vi "Thermo Analyzers Example 1.vi"() -> ()   [LabVIEW 2012]
uses:
  <vilib>/Analysis/Matrix/Datatypes/RealMatrix.ctl
  <vilib>/Analysis/Matrix/NI_Matrix.lvlib
panel:
  in  "Frequency (Hz)":dbl=0.1
  out "Data Out":T1(array[cluster])
  out "error out":errorcluster
  out "Thermo Analyzer Data":dbl[][](graph)
  in  "Stop Button":bool
  in  "Instrument":T2(ring)
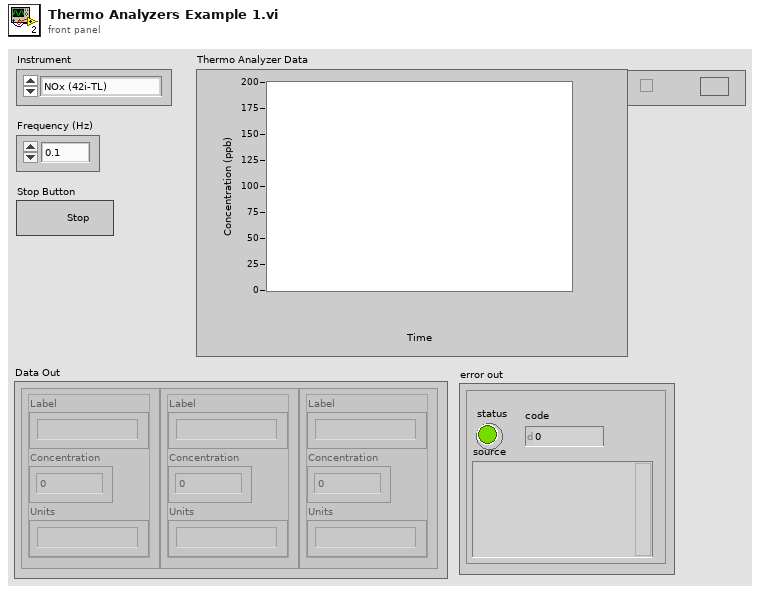
[diagram p1: front panel]
types:
  T1 = cluster{"Label":string, "Concentration":sgl, "Units":string}[]
  T2 = enum16{"NOx (42i-TL)", "SO2 (43i-TLE)", "O3 (49i)"}
  T3 = typedef "NI_Matrix.lvlib/RealMatrix.ctl" = dbl[][]
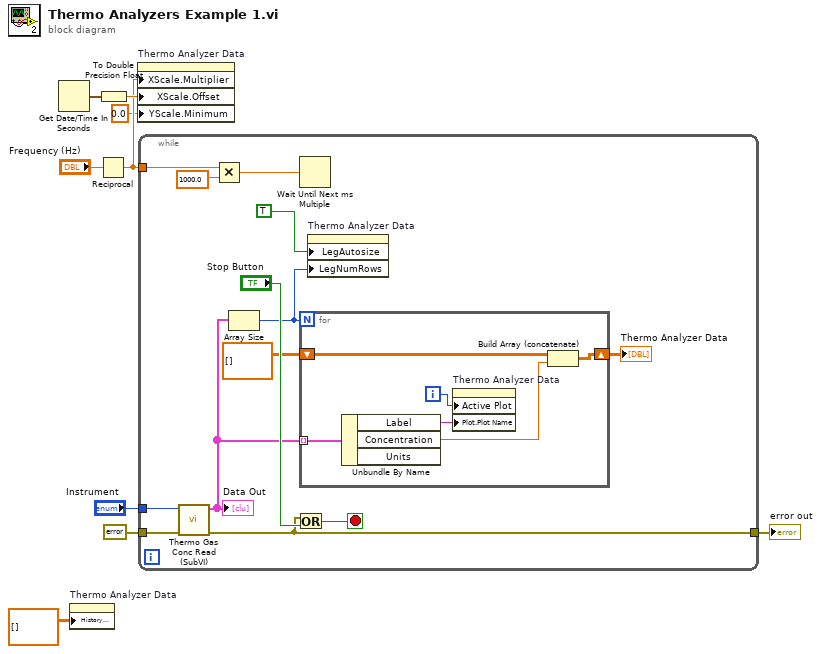
[diagram p0: block diagram]
diagram:
  n1 = Get Date/Time In Seconds() -> (seconds since 1Jan1904=w5:timestamp)
  n2 = property on="Thermo Analyzer Data" class="WFChart (strict)"("History Data"=dbl[][] []) -> ()  [unwired: 2 in, 2 out]
  n3 = Reciprocal(x="Frequency (Hz)") -> (1/x=w3:dbl)
  n4 = To Double Precision Float(number=w5) -> (double precision float=w4:dbl)
  n5 = property on="Thermo Analyzer Data" class="WFChart (strict)"("XScale.Multiplier"=w3, "XScale.Offset"=w4, "YScale.Minimum"=0.0 ("Y Scale.Range:Minimum")) -> ()  [unwired: 2 in, 2 out]
  n6 = while {
    tunnel: "Instrument" -> [w10]
    tunnel: errorcluster {"status"=FALSE, "code"=0, "source"=""} ("Error In") -> [w22]
    tunnel: [w19] -> w7
    tunnel: w3 -> [w16]
    stop <- w21 stop-if-true
    n7 = call "Thermo Gas Conc Read (SubVI).vi"("Error In"=w22, "Instrument"=w10) -> ("error out"=w19:errorcluster, "Data Out"=w13:T1)  [unwired: 8 in]
    "Data Out" <- w13
    n8 = Multiply(x=w16, y=1000.0) -> (x*y=w15:dbl)
    n9 = Array Size(array=w13) -> (size(s)=w11:i32)
    n10 = Or(x=w19, y="Stop Button") -> (x .or. y?=w21:bool)
    n11 = Wait Until Next ms Multiple(millisecond multiple=w15) -> ()  [unwired: 1 out]
    n12 = for {
      N: w11 -> [_]
      tunnel: w13 -> [w28] mode=indexing
      shift-right: [w27] -> w18
      shift-left: T3 [] ("Real Matrix") -> [w25]
      i -> [w24]
      n13 = Unbundle By Name(w28) -> ("Label"=w23:string, "Concentration"=w26:sgl)  [unwired: 1 out]
      n14 = property on="Thermo Analyzer Data" class="WFChart (strict)"("Active Plot"=w24, "Plot.Plot Name"=w23) -> ()  [unwired: 2 in, 2 out]
      n15 = Build Array (concatenate)(w25, w26) -> (w27:T3)
    }
    "Thermo Analyzer Data" <- w18
    n16 = property on="Thermo Analyzer Data" class="WFChart (strict)"("LegAutosize"=TRUE ("Legend:Autosize"), "LegNumRows"=w11) -> ()  [unwired: 2 in, 2 out]
  }
  "error out" <- w7
